vi "get Heading.vi"(11 "Motion in":refnum<class "Motion.lvclass">) -> (3 "Heading [deg]":sgl=10.0 format="%.3g")   [LabVIEW 2015, in "Motion.lvclass"]
uses:
  Motion.lvclass
  Motion.lvclass/Motion.ctl
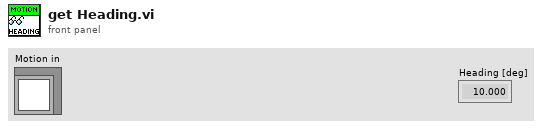
[diagram p1: front panel]
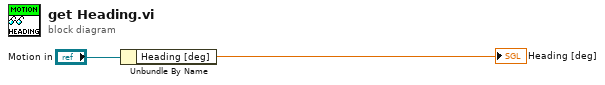
[diagram p0: block diagram]
diagram:
  n1 = Unbundle By Name("Motion in") -> ("Heading [deg]"=→"Heading [deg]":sgl)
